vi "ArmNetwork.vi"   [LabVIEW 2023]
uses:
  ArmNetworkingGlobal.vi
  <vilib>/Rock Robotics/Network Tables/NT Write Number.vi
  <vilib>/Rock Robotics/Network Tables/NT Write Boolean.vi
  ArmGlobal.vi
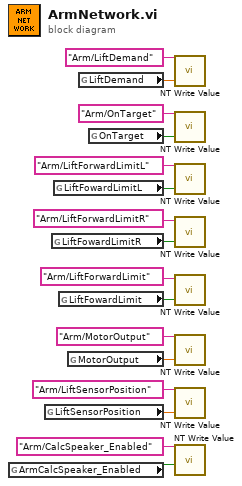
[diagram p0: block diagram]
diagram:
  n1 = global read "ArmGlobal.vi" "ArmCalcSpeaker_Enabled"() -> (w6:bool)
  n2 = global read "ArmNetworkingGlobal.vi" "LiftSensorPosition"() -> (w7:dbl)
  n3 = global read "ArmNetworkingGlobal.vi" "LiftFowardLimitR"() -> (w4:bool)
  n4 = global read "ArmNetworkingGlobal.vi" "LiftFowardLimitL"() -> (w11:bool)
  n5 = global read "ArmNetworkingGlobal.vi" "LiftFowardLimit"() -> (w2:bool)
  n6 = global read "ArmNetworkingGlobal.vi" "MotorOutput"() -> (w9:dbl)
  n7 = global read "ArmNetworkingGlobal.vi" "LiftDemand"() -> (w15:dbl)
  n8 = global read "ArmNetworkingGlobal.vi" "OnTarget"() -> (w13:bool)
  n9 = call-poly <vilib>:"NT Write Value.vi"("value"=w15, "name"="Arm/LiftDemand") -> ()  [unwired: 9 in, 1 out]
  n10 = call-poly <vilib>:"NT Write Value.vi"("value"=w13, "name"="Arm/OnTarget") -> ()  [unwired: 9 in, 1 out]
  n11 = call-poly <vilib>:"NT Write Value.vi"("value"=w11, "name"="Arm/LiftForwardLimitL") -> ()  [unwired: 9 in, 1 out]
  n12 = call-poly <vilib>:"NT Write Value.vi"("value"=w4, "name"="Arm/LiftForwardLimitR") -> ()  [unwired: 9 in, 1 out]
  n13 = call-poly <vilib>:"NT Write Value.vi"("value"=w2, "name"="Arm/LiftForwardLimit") -> ()  [unwired: 9 in, 1 out]
  n14 = call-poly <vilib>:"NT Write Value.vi"("value"=w9, "name"="Arm/MotorOutput") -> ()  [unwired: 9 in, 1 out]
  n15 = call-poly <vilib>:"NT Write Value.vi"("value"=w7, "name"="Arm/LiftSensorPosition") -> ()  [unwired: 9 in, 1 out]
  n16 = call-poly <vilib>:"NT Write Value.vi"("value"=w6, "name"="Arm/CalcSpeaker_Enabled") -> ()  [unwired: 9 in, 1 out]
